vi "AO_WriteScaledData.vi"(0 "Task ID":u32, 2 "data":dbl[](array[numeric]), 3 "error in (no error)":errorcluster, 4 "count":i32) -> (5 "Task ID":u32, 6 "remaining count":i32, 8 "error out":errorcluster)   [LabVIEW 2015]
uses:
  Windows/System32/AdvLvDaq.dll
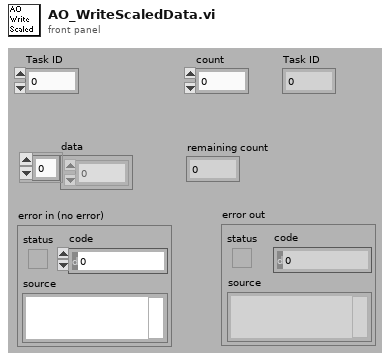
[diagram p1: front panel]
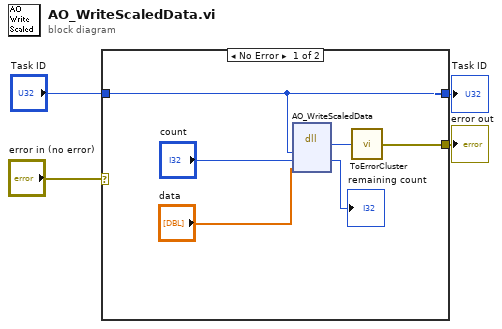
[diagram p0: block diagram]
diagram:
  n1 = case shown="No Error" "error in (no error)" {
    selector: "error in (no error)" -> [_ w11]
    tunnel: "Task ID" -> [w6 w12]
    tunnel: [w7 w11] -> w2
    tunnel: [w6 w12] -> w1
    frame No Error {
      n2 = dll-call lib="C:/Windows/System32/AdvLvDaq.dll" fn="AO_WriteScaledData"("taskId"=w6, "count"="count", "data"="data") -> ("return type"=w8:i32, "count"=→"remaining count":i32)  [unwired: 5 in, 2 out]
      n3 = call "ToErrorCluster.vi"("error code"=w8) -> ("error out"=w7:errorcluster)
    }
    frame Error {
    }
  }
  "Task ID" <- w1
  "error out" <- w2
